vi "Фильтрация показаний прибора.vi"(0 "Предпредыдущее показание":dbl, 2 "Текущее показание":dbl, 3 "Предыдущее показание":dbl, 4 "Разница между \nпоказаниями прибора":u8) -> (1 "Ошибка \nприбора":bool, 7 "Отфильтрован.\nвеличина":dbl)   [LabVIEW 2013]
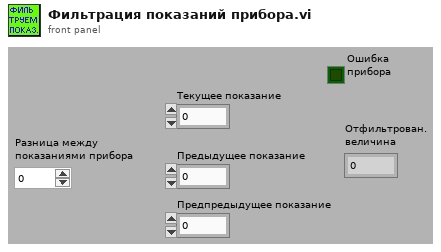
[diagram p1: front panel]
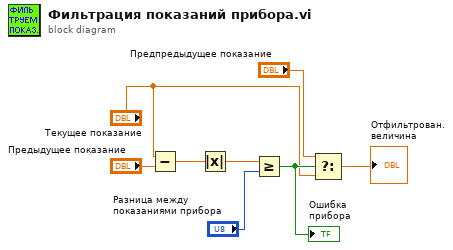
[diagram p0: block diagram]
diagram:
  n1 = Subtract(x="Текущее показание", y="Предыдущее показание") -> (x-y=w3:dbl)
  n2 = Absolute Value(x=w3) -> (abs(x)=w7:dbl)
  n3 = Greater Or Equal?(x=w7, y="Разница между \nпоказаниями прибора") -> (x >= y?=w8:bool)
  "Ошибка \nприбора" <- w8
  n4 = Select(t="Предпредыдущее показание", s=w8, f="Текущее показание") -> (s? t:f=→"Отфильтрован.\nвеличина":dbl)
